vi "Write Groups.vi"(8 "error in (no error)":errorcluster, 10 "Groups":T1(array[cluster]), 11 "ParseSVG in":refnum<class "ParseSVG.lvclass">) -> (0 "error out":errorcluster, 3 "ParseSVG out":refnum<class "ParseSVG.lvclass">)   [LabVIEW 2019, in "ParseSVG.lvclass"]
uses:
  ParseSVG.lvclass
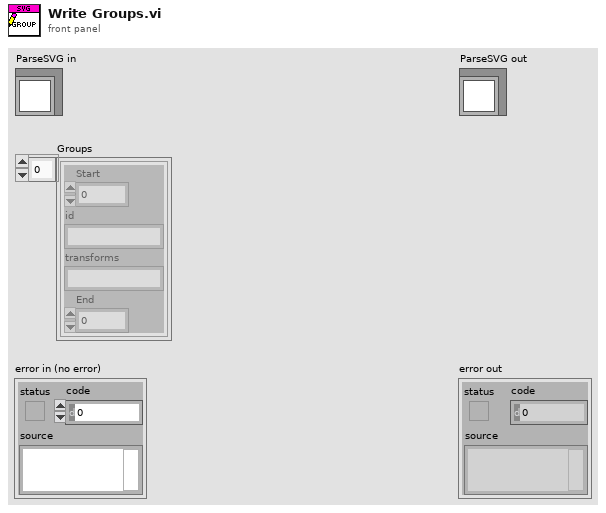
[diagram p1: front panel]
types:
  T1 = cluster{"Start":i32, "id":string, "transforms":string, "End":i32}[]
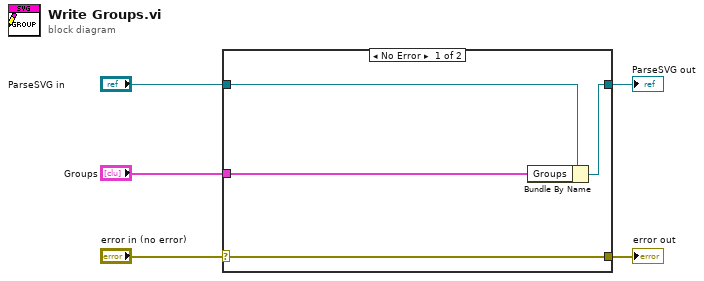
[diagram p0: block diagram]
diagram:
  n1 = case shown="No Error" "error in (no error)" {
    selector: "error in (no error)" -> [w9 w10]
    tunnel: [w9 w10] -> w4
    tunnel: [w7 w11] -> w2
    tunnel: "ParseSVG in" -> [w8 w11]
    tunnel: "Groups" -> [w6 _]
    frame No Error {
      n2 = Bundle By Name(cluster=w8, "Groups"=w6) -> (w7:refnum<class "ParseSVG.lvclass">)
    }
    frame Error {
    }
  }
  "error out" <- w4
  "ParseSVG out" <- w2
